vi "mag-field_set-coil-current.vi"(8 "mode":T1=0.12 items=["12A"=0.012, "120A"=0.12], 10 "Current (A)":dbl min=0.0 max=120.0, 11 "GPIB adr in":string="0:1") -> (3 "GPIB adr out":string="0:1")   [LabVIEW 2010]
uses:
  mode (120A-12A).ctl
panel:
  # "Input a double with the actual curernt you wish"
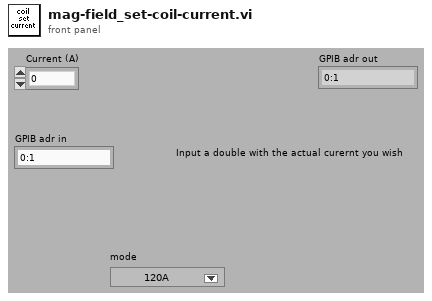
[diagram p1: front panel]
types:
  T1 = typedef "mode (120A-12A).ctl" = dbl
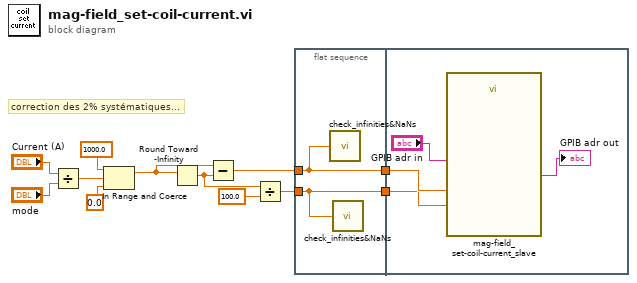
[diagram p0: block diagram]
diagram:
  # "correction des 2% systématiques..."
  n1 = Divide(x="Current (A)", y="mode") -> (x/y=w10:T1)
  n2 = In Range and Coerce(upper limit=1000.0, x=w10, lower limit=0.0) -> (coerced(x)=w8:T1)  [unwired: 1 out]
  n3 = Round Toward -Infinity(1:w8) -> (0:w6:T1)
  n4 = Subtract(x=w8, y=w6) -> (x-y=w4:T1)
  n5 = Divide(x=w6, y=100.0 ("x")) -> (x/y=w3:T1)
  n6 = flat-sequence {
    tunnel: w3 -> [w14]
    tunnel: w4 -> [w13]
    tunnel: [w13] -> w2
    tunnel: [w14] -> w1
    tunnel: w2 -> [w18]
    tunnel: w1 -> [w17]
    frame #0 {
      n7 = call "check_infinities&NaNs.vi"("Value"=w13) -> ()
      n8 = call "check_infinities&NaNs.vi"("Value"=w14) -> ()
    }
    frame #1 {
      n9 = call "mag-field_set-coil-current_slave.vi"("GPIB adr in"="GPIB adr in", "Current (100% scale)"=w17, "current (1% scale)"=w18) -> ("GPIB adr out"=→"GPIB adr out":string)  [unwired: 24 out]
    }
  }
